vi "ex2_1.vi"() -> ()   [LabVIEW 2017]
uses:
  <vilib>/measure/NI_MABase.lvlib
panel:
  out "Waveform Graph":dynamicdata(graph)
  out "Sin":bool
  in  "Saw tooth":bool
  in  "Triangular":bool
  in  "Square":bool
  in  "Sin":bool
  out "Saw tooth":bool
  out "Triangular":bool
  out "Square":bool
  in  "Ampiude":dbl
  in  "Frequency":dbl
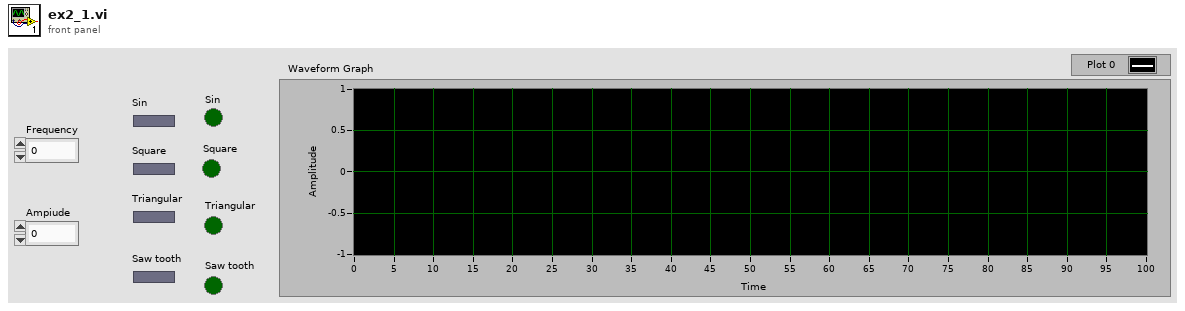
[diagram p1: front panel]
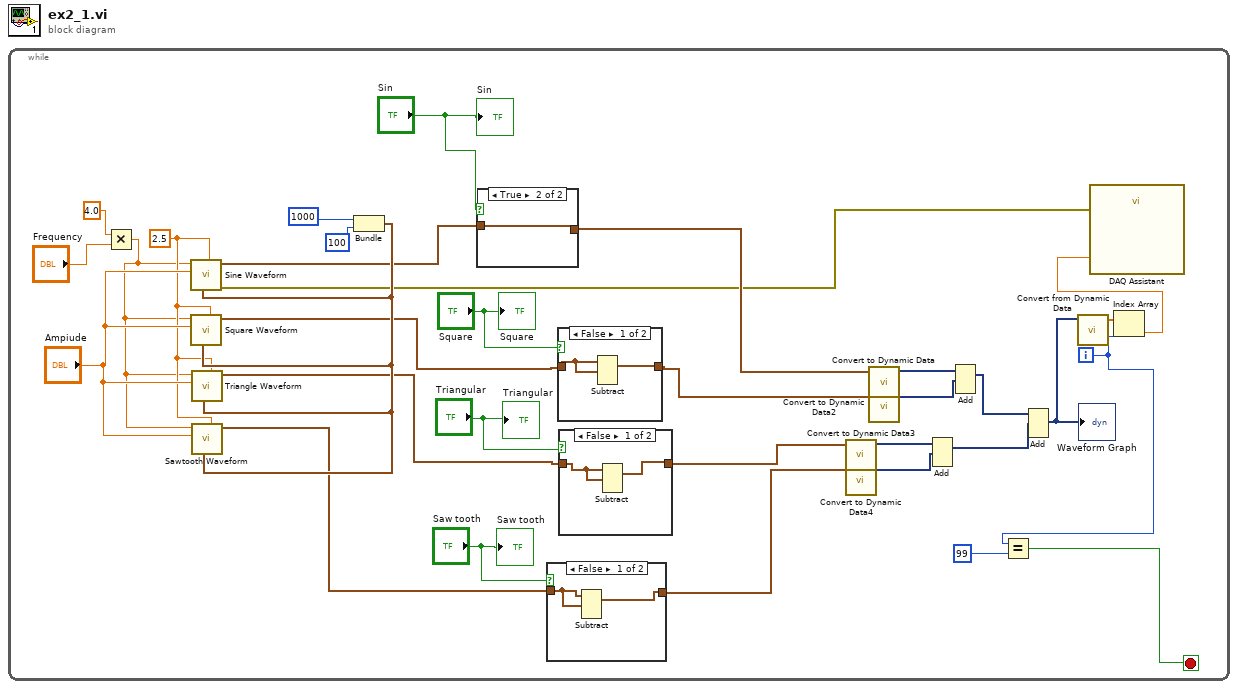
[diagram p0: block diagram]
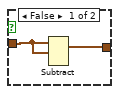
[diagram p5: hidden frame]
diagram:
  n1 = while {
    i -> [w4]
    stop <- w6 stop-if-true
    w11 = 2.5
    n2 = Multiply(x=4.0, y="Frequency") -> (x*y=w2:dbl)
    n3 = Bundle(1000, 100) -> (w32:cluster{i32, i32})  [unwired: 1 in]
    n4 = call <vilib>:"Sine Waveform.vi"("offset"=w11, "sampling info"=w32, "amplitude"="Ampiude", "frequency"=w2) -> ("error out"=w12:errorcluster, "signal out"=w31:waveform(dbl))  [unwired: 6 in]
    n5 = call <vilib>:"Square Waveform.vi"("offset"=w11, "sampling info"=w32, "amplitude"="Ampiude", "frequency"=w2) -> ("signal out"=w28:waveform(dbl))  [unwired: 6 in, 1 out]
    n6 = call <vilib>:"Triangle Waveform.vi"("offset"=w11, "sampling info"=w32, "amplitude"="Ampiude", "frequency"=w2) -> ("signal out"=w26:waveform(dbl))  [unwired: 6 in, 1 out]
    n7 = call <vilib>:"Sawtooth Waveform.vi"("offset"=w11, "sampling info"=w32, "amplitude"="Ampiude", "frequency"=w2) -> ("signal out"=w24:waveform(dbl))  [unwired: 6 in, 1 out]
    n8 = case shown="True" "Sin" {
      tunnel: w31 -> [w44 w45]
      tunnel: [w43 w45] -> w23
      frame False {
        n9 = Subtract(1:w44, 2:w44) -> (0:w43:waveform(dbl))  [unwired: 1 in, 1 out]
      }
      frame True {
      }
    }
    n10 = case shown="False" "Saw tooth" {
      tunnel: w24 -> [w35 w36]
      tunnel: [w34 w36] -> w17
      frame False {
        n11 = Subtract(1:w35, 2:w35) -> (0:w34:waveform(dbl))  [unwired: 1 in, 1 out]
      }
      frame True {
      }
    }
    n12 = case shown="False" "Square" {
      tunnel: w28 -> [w41 w42]
      tunnel: [w40 w42] -> w19
      frame False {
        n13 = Subtract(1:w41, 2:w41) -> (0:w40:waveform(dbl))  [unwired: 1 in, 1 out]
      }
      frame True {
      }
    }
    n14 = case shown="False" "Triangular" {
      tunnel: w26 -> [w38 w39]
      tunnel: [w37 w39] -> w18
      frame False {
        n15 = Subtract(1:w38, 2:w38) -> (0:w37:waveform(dbl))  [unwired: 1 in, 1 out]
      }
      frame True {
      }
    }
    n16 = call "Convert to Dynamic Data3"("Array"=w18) -> ("Dynamic Data Type"=w21:dynamicdata)  [unwired: 3 in]
    n17 = call "Convert to Dynamic Data4"("Array"=w17) -> ("Dynamic Data Type"=w20:dynamicdata)  [unwired: 3 in]
    n18 = call "Convert to Dynamic Data"("Array"=w23) -> ("Dynamic Data Type"=w13:dynamicdata)  [unwired: 3 in]
    n19 = call "Convert to Dynamic Data2"("Array"=w19) -> ("Dynamic Data Type"=w22:dynamicdata)  [unwired: 3 in]
    n20 = Add(1:w20, 2:w21) -> (0:w16:dynamicdata)  [unwired: 1 in, 1 out]
    n21 = Add(1:w22, 2:w13) -> (0:w15:dynamicdata)  [unwired: 1 in, 1 out]
    n22 = Equal?(x=w4, y=99) -> (x = y?=w6:bool)
    n23 = Add(1:w16, 2:w15) -> (0:w5:dynamicdata)  [unwired: 1 in, 1 out]
    "Waveform Graph" <- w5
    n24 = call "Convert from Dynamic Data"("Dynamic Data Type"=w5) -> ("Array"=w14:dbl[])  [unwired: 3 in]
    n25 = Index Array(array=w14, index=w4) -> (element=w8:dbl)
    n26 = call "DAQ Assistant"("data"=w8, "error in"=w12) -> ()  [unwired: 16 in, 2 out]
    "Square" <- "Square"
    "Triangular" <- "Triangular"
    "Saw tooth" <- "Saw tooth"
    "Sin" <- "Sin"
  }
